vi "Review Result.vi"(0 "Vector 26GHz Path in":refnum<class "Vector Path.lvclass">, 11 "error in (no error)":errorcluster) -> (4 "Vector 26GHz Path out":refnum<class "Vector Path.lvclass">, 6 "Response":string, 15 "error out":errorcluster)   [LabVIEW 2023, in "RFFixtureCharact.Public.lvlib" / "Vector Path.lvclass"]
uses:
  Vector Path.lvclass
  C:/rfcal/AuxTools/STSRFFixtureCharactUtility/Source/Code Modules/Common/Base Classes/Path/Path.lvclass
  Vector Abstract Path/Type Definitions/Vector Charact Result.ctl
  <vilib>/Utility/error.llb/Trim Whitespace One-Sided.vi
  Vector Path.lvclass/Vector Path.ctl
  Vector Abstract Path/Vector Abstract Path.lvclass
  Common/RFCalAndFixtureCharact.Common.lvlib
  RFFixtureCharact.Public.lvlib
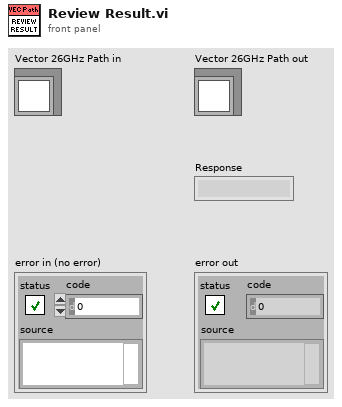
[diagram p1: front panel]
types:
  T1 = typedef "RFFixtureCharact.Public.lvlib/Vector Abstract Path.lvclass/Vector Charact Result.ctl" = cluster{"Port Power":dbl, "Frequency":dbl, "S Parameters":cdb[], "Out Of Limit":bool}
  T2 = typedef "RFFixtureCharact.Public.lvlib/Vector Path Group.lvclass/Sweep.ctl" = cluster{"Port Power":dbl, "Frequencies":dbl[], "Test Receiver Attenuation":dbl, "IF Bandwidth":dbl}
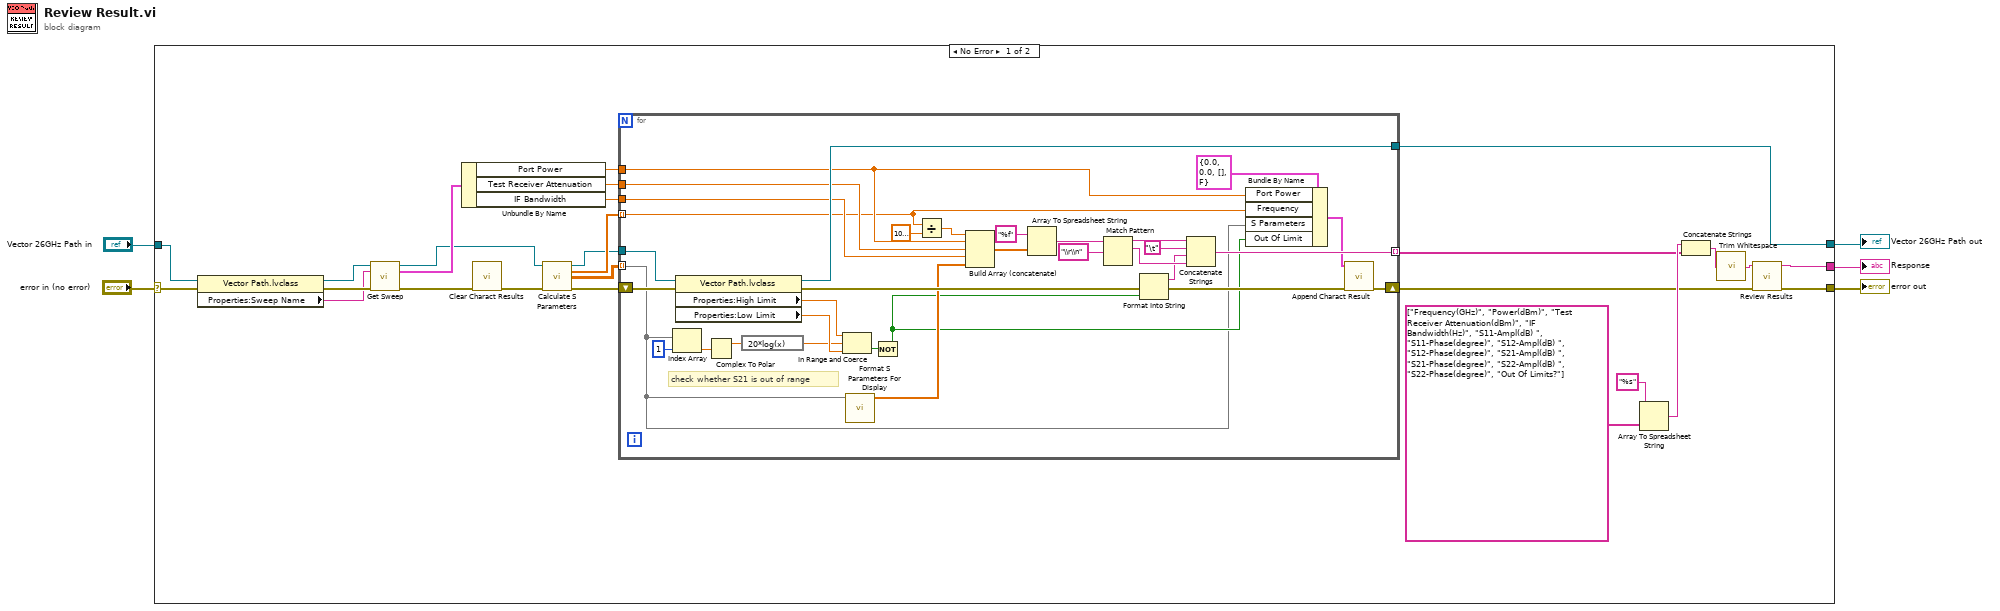
[diagram p0: block diagram]
diagram:
  n1 = case shown="No Error" "error in (no error)" {
    selector: "error in (no error)" -> [w29 w66]
    tunnel: [w26 w65] -> w1
    tunnel: [w27 _] -> w2
    tunnel: [w28 w66] -> w3
    tunnel: "Vector 26GHz Path in" -> [w31 w65]
    frame No Error {
      n2 = property class="Vector Path.lvclass"(reference=w31, error in=w29) -> (reference out=w7:refnum<class "Vector Path.lvclass">, error out=w30:errorcluster, "Properties:Sweep Name"=w9:string)
      n3 = call-dynamic "Get Sweep.vi"("Vector Path in"=w7, "Sweep Name"=w9, "error in (no error)"=w30) -> ("Vector Path out"=w6:refnum<class "Vector Path.lvclass">, "Sweep"=w8:T2, "error out"=w11:errorcluster)  [unwired: 9 in, 1 out]
      n4 = Unbundle By Name(w8) -> ("Port Power"=w24:dbl, "Test Receiver Attenuation"=w25:dbl, "IF Bandwidth"=w12:dbl)
      n5 = call "Clear Charact Results.vi"("error in"=w11) -> ("error out"=w10:errorcluster)  [unwired: 14 in]
      n6 = call-dynamic "Calculate S Parameters.vi"("Vector Path in"=w6, "error in (no error)"=w10) -> ("Vector Path out"=w14:refnum<class "Vector Path.lvclass">, "Frequencies"=w23:dbl[], "S Parameters out"=w22:cdb[][], "error out"=w13:errorcluster)  [unwired: 10 in]
      n7 = for {
        shift-right: [w35] -> w16
        shift-left: w13 -> [w64]
        tunnel: w23 -> [w37] mode=indexing
        tunnel: w22 -> [w32] mode=indexing
        tunnel: w14 -> [w63]
        tunnel: w25 -> [w44]
        tunnel: w24 -> [w38]
        tunnel: [w55] -> w26
        tunnel: [w42] -> w15 mode=indexing
        tunnel: w12 -> [w41]
        # "check whether S21 is out of range"
        n8 = Index Array(array=w32, index=1) -> (element=w61:cdb)
        n9 = property class="Vector Path.lvclass"(reference=w63, error in=w64) -> (reference out=w55:refnum<class "Vector Path.lvclass">, error out=w43:errorcluster, "Properties:High Limit"=w59:dbl, "Properties:Low Limit"=w58:dbl)
        n10 = Complex To Polar(r * e^(i*theta)=w61) -> (r=w57:dbl)  [unwired: 1 out]
        n11 = expression code="20*log(x)"(w57) -> (w56:dbl)
        n12 = In Range and Coerce(upper limit=w59, x=w56, lower limit=w58) -> (In Range?=w60:bool)  [unwired: 1 out]
        n13 = call "Format S Parameters For Display.vi"("S Parameters"=w32) -> ("S Parameters For Display"=w34:dbl[])  [unwired: 14 in]
        n14 = Not(x=w60) -> (.not. x?=w33:bool)
        n15 = Divide(x=w37, y=1000000000.0) -> (x/y=w53:dbl)
        n16 = Build Array (concatenate)(w53, w38, w44, w41, w34) -> (w49:dbl[])
        n17 = Array To Spreadsheet String(array=w49, 3:"%f" ("format string")) -> (spreadsheet string=w51:string)  [unwired: 1 in]
        n18 = Match Pattern(string=w51, regular expression="\\r\\n") -> (before substring=w48:string, match substring=w46:string)  [unwired: 1 in, 2 out]
        n19 = Format Into String(error in=w43, w33) -> (resulting string=w45:string, error out=w36:errorcluster)  [unwired: 2 in]
        n20 = Concatenate Strings(w48, "\t", w45, w46) -> (w42:string)
        n21 = Bundle By Name(cluster=T1 {"Port Power"=0.0, "Frequency"=0.0, "S Parameters"=[], "Out Of Limit"=FALSE} ("Charact Result"), "Port Power"=w38, "Frequency"=w37, "S Parameters"=w32, "Out Of Limit"=w33) -> (w39:T1)
        n22 = call "Append Charact Result.vi"("Path cal resut in"=w39, "error in (no error)"=w36) -> ("error out"=w35:errorcluster)  [unwired: 13 in]
      }
      n23 = Array To Spreadsheet String(array=string[] ["Frequency(GHz)", "Power(dBm)", "Test Receiver Attenuation(dBm)", "IF Bandwidth(Hz)", "S11-Ampl(dB) ", "S11-Phase(degree)", "S12-Ampl(dB) ", "S12-Phase(degree)", "S21-Ampl(dB) ", "S21-Phase(degree)", "S22-Ampl(dB) ", "S22-Phase(degree)", "Out Of Limits?"], 3:"%s" ("format string")) -> (spreadsheet string=w19:string)  [unwired: 1 in]
      n24 = Concatenate Strings(w19, w15) -> (w18:string)
      n25 = call <vilib>:"Trim Whitespace.vi"("string"=w18) -> ("trimmed string"=w17:string)  [unwired: 1 in]
      n26 = call "Review Results.vi"("Cal Results"=w17, "error in (no error)"=w16) -> ("Response"=w27:string, "error out"=w28:errorcluster)  [unwired: 12 in]
    }
    frame Error {
    }
  }
  "error out" <- w3
  "Vector 26GHz Path out" <- w1
  "Response" <- w2
